vi "LINC Scan Tokens.vi"(1 "string":string) -> (0 "tokens":string[](array[string]))   [LabVIEW 2018, in "STEPkgDriver_LINC.lvlib"]
uses:
  STEPkgDriver_LINC.lvlib
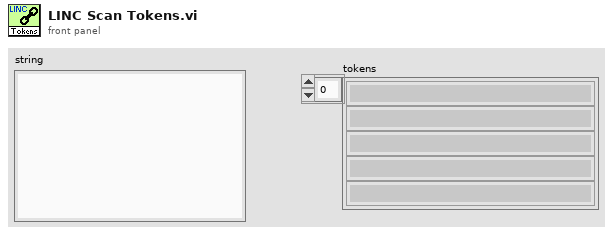
[diagram p1: front panel]
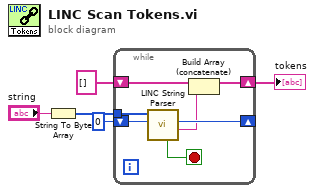
[diagram p0: block diagram]
diagram:
  n1 = String To Byte Array(string="string") -> (unsigned byte array=w4:u8[])
  n2 = while {
    shift-right: [w10] -> _
    shift-left: 0 ("index out") -> [w11]
    tunnel: w4 -> [w12]
    shift-right: [w7] -> w1
    shift-left: string[] [] -> [w8]
    stop <- w9 stop-if-true
    n3 = call "LINC String Parser.vi"("index in"=w11, "string in"=w12) -> ("string found"=w6:string, "index out"=w10:i32, "end"=w9:bool)  [unwired: 5 in, 2 out]
    n4 = Build Array (concatenate)(w8, w6) -> (w7:string[])
  }
  "tokens" <- w1
